vi "Connect.vi"(8 "error in (no error)":errorcluster, 11 "PXI6521 in":refnum<class "PXI6521.lvclass">) -> (0 "error out":errorcluster, 3 "PXI6521 out":refnum<class "PXI6521.lvclass">)   [LabVIEW 2018, in "PXI6521.lvlib" / "PXI6521.lvclass"]
uses:
  PXI6521.lvclass
  PPLs/DigitalIO/Parent/DigitalIO.lvlibp/DigitalIO.lvclass
  C:/Projects/LabVIEW/PPLs/DigitalIO/Parent/DigitalIO.lvlibp/DigitalIO.lvclass
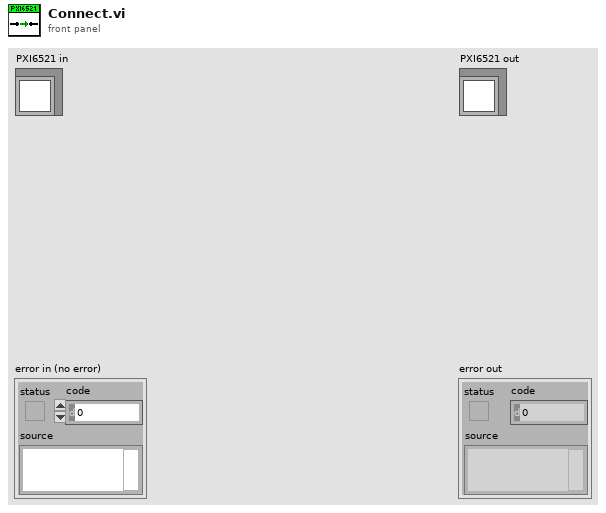
[diagram p1: front panel]
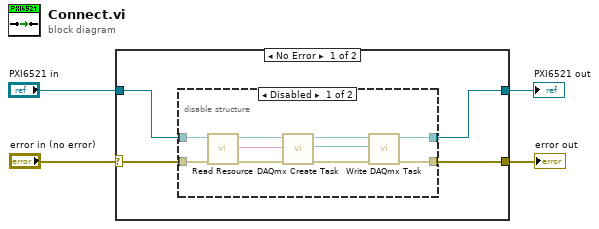
[diagram p0: block diagram]
diagram:
  n1 = case shown="No Error" "error in (no error)" {
    selector: "error in (no error)" -> [w8 w21]
    tunnel: [w6 w21] -> w3
    tunnel: [w5 w20] -> w2
    tunnel: "PXI6521 in" -> [w7 w20]
    frame No Error {
      n2 = disable-structure shown="Disabled" {
        disable-tunnel: w8 -> [w17 w18]
        disable-tunnel: w7 -> [w16 w19]
        disable-tunnel: [w15 w18] -> w6
        disable-tunnel: [w14 w19] -> w5
        frame Disabled {
          n3 = call "Read Resource.vi"("error in (no error)"=w17, "DigitalIO in"=w16) -> ("error out"=w13:errorcluster, "Resource"=w12:string, "DigitalIO out"=w9:refnum<class "PXI6521.lvclass">)  [unwired: 7 in]
          n4 = call <vilib>:"DAQmx Create Task.vi"("new task name"=w12, "error in"=w13) -> ("task out"=w10:refnum<k21>, "error out"=w11:errorcluster)  [unwired: 12 in]
          n5 = call "Write DAQmx Task.vi"("error in (no error)"=w11, "DAQmx Task"=w10, "PXI6521 in"=w9) -> ("error out"=w15:errorcluster, "PXI6521 out"=w14:refnum<class "PXI6521.lvclass">)  [unwired: 7 in]
        }
        frame Enabled {
        }
      }
    }
    frame Error {
    }
  }
  "error out" <- w3
  "PXI6521 out" <- w2
